vi "XY曲线.vi"(9 "动作":enum16{"读取", "添加", "删除"}(ring), 10 "y":dbl[](array[numeric]), 11 "x":dbl[](array[numeric])) -> (3 "数组":cluster{"x":dbl[], "y":dbl[]}[](array[cluster]))   [LabVIEW 2015]
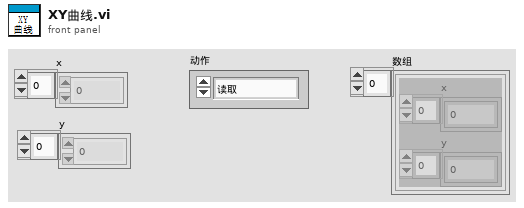
[diagram p1: front panel]
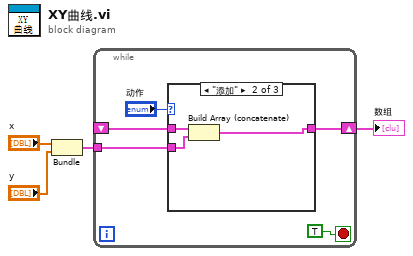
[diagram p0: block diagram]
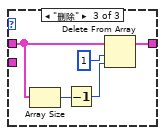
[diagram p3: hidden frame]
diagram:
  n1 = Bundle("x"="x", "y"="y") -> (w2:cluster{"x":dbl[], "y":dbl[]})  [unwired: 1 in]
  n2 = while {
    shift-right: [w7] -> w1
    shift-left: _ -> [w6]
    tunnel: w2 -> [w8]
    stop <- TRUE stop-if-true
    n3 = case shown="\"添加\"" "动作" {
      tunnel: w8 -> [_ w13 _]
      tunnel: [w10 w12 w14] -> w7
      tunnel: w6 -> [w10 w11 w17]
      frame "读取", Default {
      }
      frame "添加" {
        n4 = Build Array (concatenate)(w11, w13) -> (w12:cluster{"x":dbl[], "y":dbl[]}[])
      }
      frame "删除" {
        n5 = Array Size(array=w17) -> (size(s)=w16:i32)
        n6 = Decrement(x=w16) -> (x-1=w15:i32)
        n7 = Delete From Array(array=w17, length=1 ("长度"), index=w15) -> (array with subset deleted=w14:cluster{"x":dbl[], "y":dbl[]}[])  [unwired: 1 out]
      }
    }
  }
  "数组" <- w1
